vi "Testing FFT.vi"() -> ()   [LabVIEW 2012]
uses:
  <vilib>/Analysis/2dsp.llb/Inverse Real FFT.vi
  <vilib>/express/express analysis/Spectral/Block/exnSpectralBlock spectral measurements RMS poly.vi
  <vilib>/express/express analysis/Spectral/Block/exnSpectralBlock spectral measurements RMS DDT.vi
  <vilib>/express/express analysis/Spectral/XNode/ExpressSpectralMeasurementsBlockNode.xnode
  <vilib>/Analysis/NI_AALPro.lvlib
panel:
  out "Waveform Graph 2":dynamicdata(graph)
  out "XY Graph":cluster{"X":dbl, "Y":dbl}[](graph)
  out "XY Graph 2":cluster{"X":dbl, "Y":dbl}[](graph)
  out "Frequency":dbl
  out "Amplitude":dbl
  out "Waveform Graph":dbl[](graph)
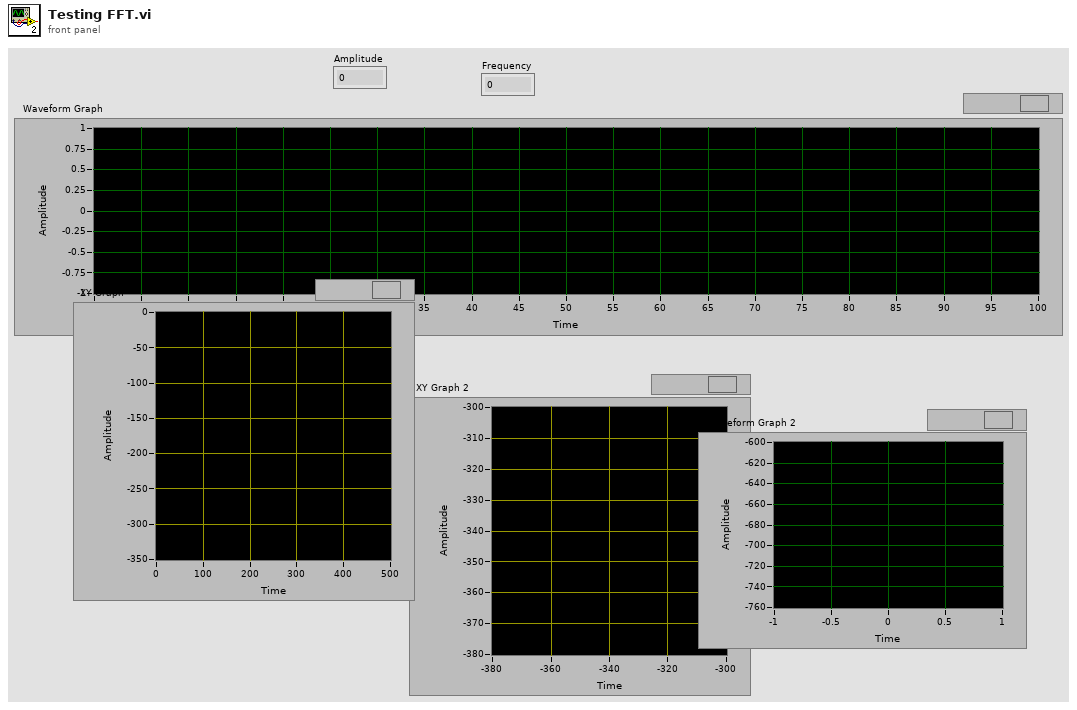
[diagram p1: front panel]
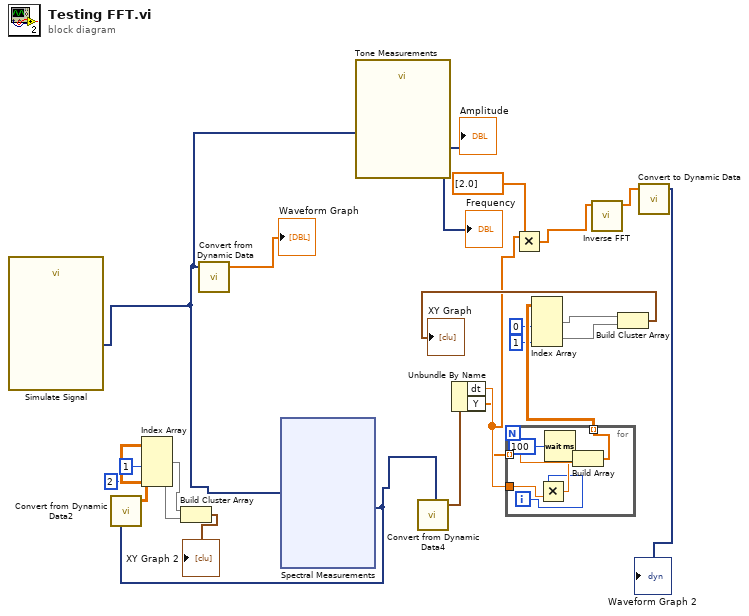
[diagram p0: block diagram]
diagram:
  n1 = call "Simulate Signal"() -> ("Square"=w20:dynamicdata)  [unwired: 14 in, 1 out]
  n2 = call "Convert from Dynamic Data"("Dynamic Data Type"=w20) -> ("Array"=→"Waveform Graph":dbl[])  [unwired: 3 in]
  n3 = xnode "Spectral Measurements"("Signals"=w20) -> ("FFT - (RMS)"=w19:dynamicdata)  [unwired: 1 in, 2 out]
  n4 = call "Convert from Dynamic Data2"("Dynamic Data Type"=w19) -> ("Array"=w18:dbl[][])  [unwired: 3 in]
  n5 = Index Array(array=w18, index (col) #1=1 ("disabled index (col)"), index (col) #2=2 ("index (col)")) -> (element #1=w17:dbl[], element #2=w16:dbl[])  [unwired: 2 in]
  n6 = Build Cluster Array(w17, w16) -> (→"XY Graph 2":cluster{"element":dbl, "element":dbl}[])
  n7 = call "Tone Measurements"("Signals"=w20) -> ("Frequency"=→"Frequency":dynamicdata, "Amplitude"=→"Amplitude":dynamicdata)  [unwired: 8 in, 1 out]
  n8 = call "Convert from Dynamic Data4"("Dynamic Data Type"=w19) -> ("Waveform"=w21:waveform(dbl))  [unwired: 3 in]
  n9 = Unbundle By Name(w21) -> ("dt"=w12:dbl, "Y"=w5:dbl[])
  n10 = for {
    tunnel: w12 -> [w27]
    tunnel: w5 -> [w30] mode=indexing
    tunnel: [w28] -> w11 mode=indexing
    i -> [w26]
    n11 = Multiply(x=w26, y=w27) -> (x*y=w29:dbl)
    n12 = Wait (ms)(milliseconds to wait=u32 100) -> ()  [unwired: 1 out]
    n13 = Build Array(w29, w30) -> (w28:dbl[])
  }
  n14 = Multiply(x=w5, y=dbl[] [2.0]) -> (x*y=w3:dbl[])
  n15 = Index Array(array=w11, index (col) #1=0 ("disabled index (col)"), index (col) #2=1 ("index (col)")) -> (element #1=w8:dbl[], element #2=w7:dbl[])  [unwired: 2 in]
  n16 = call-poly <vilib>:"Inverse FFT.vi"("FFT {X}"=w3) -> ("X"=w2:dbl[])  [unwired: 9 in, 1 out]
  n17 = Build Cluster Array(w8, w7) -> (→"XY Graph":cluster{dbl, dbl}[])
  n18 = call "Convert to Dynamic Data"("Array"=w2) -> ("Dynamic Data Type"=→"Waveform Graph 2":dynamicdata)  [unwired: 3 in]
